vi "getConversionFactorCluster.vi"(7 "error in (no error)":errorcluster, 10 "Protocol_Logging in":refnum<class "Protocol_Logging.lvclass">) -> (0 "error out":errorcluster, 2 "conversionFactorCluster":T1, 3 "Protocol_Logging out":refnum<class "Protocol_Logging.lvclass">)   [LabVIEW 2011, in "Protocol_Logging.lvclass"]
uses:
  Protocol_Logging.lvclass
  Protocol_Logging.lvclass/Protocol_Logging.ctl
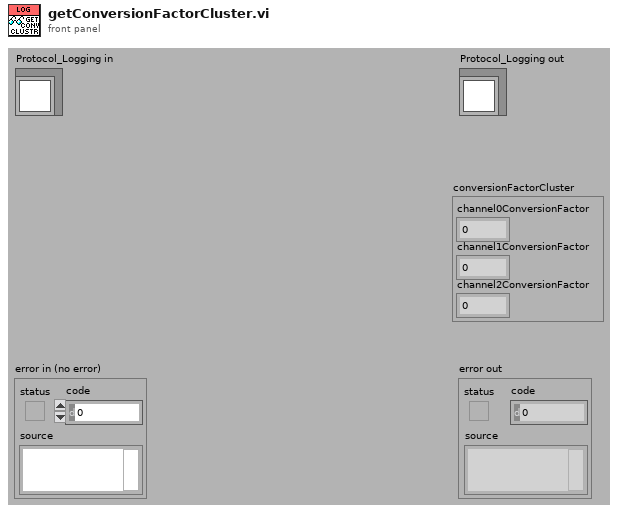
[diagram p1: front panel]
types:
  T1 = cluster{"channel0ConversionFactor":dbl, "channel1ConversionFactor":dbl, "channel2ConversionFactor":dbl}
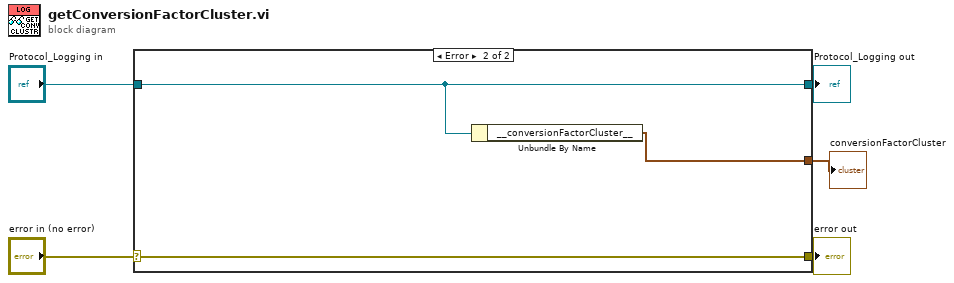
[diagram p0: block diagram]
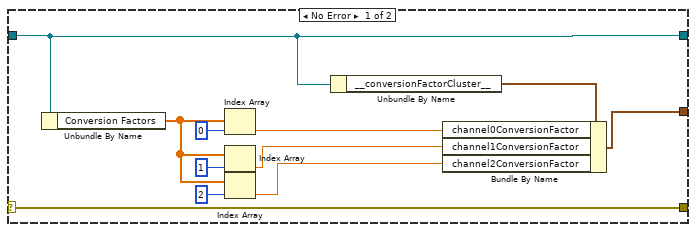
[diagram p2: hidden frame]
diagram:
  n1 = case shown="Error" "error in (no error)" {
    selector: "error in (no error)" -> [w16 w19]
    tunnel: [w16 w19] -> w4
    tunnel: [w15 w18] -> w2
    tunnel: "Protocol_Logging in" -> [w15 w18]
    tunnel: [w13 w17] -> w1
    frame No Error {
      n2 = Unbundle By Name(w15) -> ("Conversion Factors"=w8:dbl[])
      n3 = Index Array(array=w8, index=0) -> (element=w11:dbl)
      n4 = Index Array(array=w8, index=1) -> (element=w7:dbl)
      n5 = Index Array(array=w8, index=2) -> (element=w6:dbl)
      n6 = Unbundle By Name(w15) -> ("__conversionFactorCluster__"=w14:T1)
      n7 = Bundle By Name(cluster=w14, "channel0ConversionFactor"=w11, "channel1ConversionFactor"=w7, "channel2ConversionFactor"=w6) -> (w13:T1)
    }
    frame Error {
      n8 = Unbundle By Name(w18) -> ("__conversionFactorCluster__"=w17:T1)
    }
  }
  "error out" <- w4
  "Protocol_Logging out" <- w2
  "conversionFactorCluster" <- w1
